vi "global constants.vi"() -> ()   [LabVIEW 2016, in "FPGA Resource Manager.lvlib"]
uses:
  FPGA Resource Manager.lvlib
panel:
  in  "Tags":enum32{"Client", "Server", "Shared"}(tab)=enum."Server"
  in  "Client":string="RM.Client"
  in  "max column width":i32=400
  in  "character size":i32=7
  in  "viz.sidebar.max":i32=270
  in  "viz.sidebar.min":i32=30
  in  "Reservation Format String":string="RM.Reservation.%s"
  in  "Server":string="RM.Server"
  in  "Visualizer Status":string="rm.visualizer.status"
  in  "Sort Types":string[](array[string])=["FPGA CD", "resource", "input type", "datatype", "reserver", "notes"]
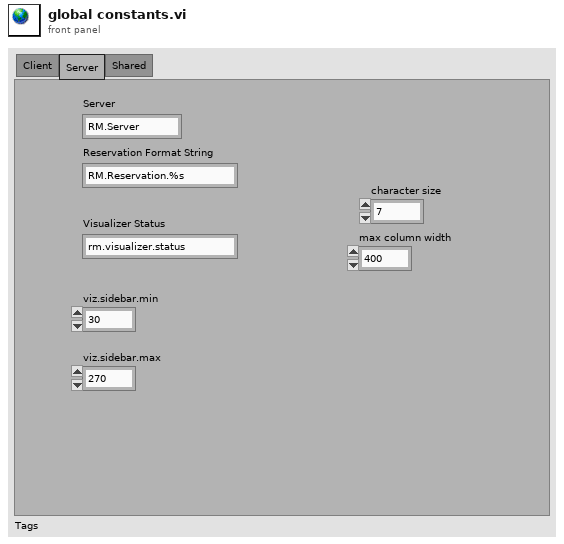
[diagram p1: front panel]
diagram:
